vi "EventLog.New(single).vi"(7 "Source (All)":T1, 8 "error in (no error)":errorcluster, 9 "Arg":variant, 10 "Message (-)":T2, 11 "Level (Info)":T3=enum."Info") -> (0 "error out":errorcluster, 2 "Translated Msg":string)   [LabVIEW 2016]
uses:
  EventLog.EventLevel.ctl
  Translator/Translator.Message.ctl
  EventLog.EventSource.ctl
  EventLog.EventGui.ctl
  EventLog.Event.ctl
  EventLog.Buffer.Action.ctl
  Global/ApplicationGlobal.vi
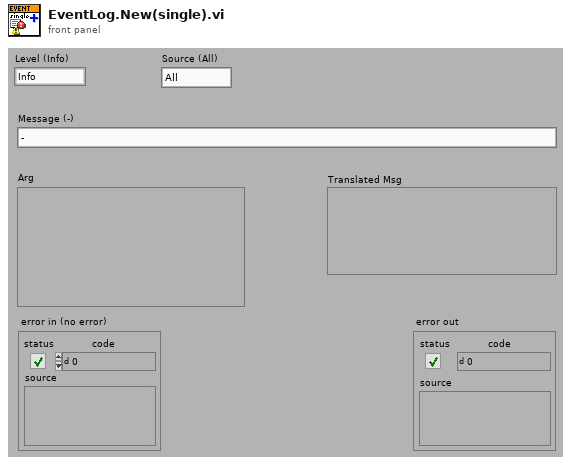
[diagram p1: front panel]
types:
  T1 = typedef "EventLog.EventSource.ctl" = enum16{"All", "Gui", "Cache", "PLC1", "PLC2", "PLC3", "DB", "DB01", "DB02", "DB03", "DB04", "DB05", "DB06", "DB07", "DB08", "DB09", "DB10", "DB11", "DB12", "DB13", "DB14", "DB15", "DB16"}
  T2 = typedef "Translator.Message.ctl" = enum16{"-", "Event confirmed", "Log out", "Log in", "Shutdown", "Cancel", "Start", "Continue", "Stop", "On", "Off", "OK", "NOK", "NOK %s", "This", "Prev", "Home", "Work", "In progress...", "Missing", "Empty", "Hardware failure", "Initial", "Error %d >> %s", "Error %d >> %s >> %s", "Starting %s", "Quitting %s", "Configured", "Initializing", "Quitting", "Loading", "Running %s", "Stopped", "Summary", "Do you want to continue?", "Do you want to exit?", "Log out?", "System", "All", "IDLE", "Translating...%s", "Not found", "Alarm %s", "Run", "Skip", "Abort", "Repeat", "Please wait...", "Database disconnected", "Login to database successful", "Login to database failed: %d; %s", "Get process step data for %s", "Changeover off", "Changeover into %s", "Product %s | %s found in cache with status %d at previous station", "Product %s | %s found in database with status %d at previous station", "Product %s | %s not found in cache at previous station", "Product %s | %s not found in database at previous station", "Product %s | %s found in cache with status %d at this station (%d repetion)", "Product %s | %s found in database with status %d at this station (%d repetition)", "Product %s | %s not found in cache at this station", "Product %s | %s not found in database at this station", "Product %s | %s found in cache for component %s | %s", "Product %s | %s found in database for component %s | %s", "Product not found in cache for component %s | %s", "Product not found in database for component %s | %s", "Product %s | %s connected with component %s | %s (cache)", "Product %s | %s connected with component %s | %s (database)", "New data for %s | %s (cache)", "New data for %s | %s (database)", "File %s moved (cache)", "File %s deleted (cache)", "Msg %d >> %s", "PLC LifeBit Failure", "Reconnecting DB", "Reconnecting PLC", "Free disk space is below 1GB - contact technician", "Unable to check product status", "Product %s SN %s checked in DB", "Unable To check status from station %s"}
  T3 = typedef "EventLog.EventLevel.ctl" = enum8{"Debug", "Info", "Warning", "Error"}
  T4 = typedef "EventLog.Event.ctl" = cluster{"ts":dbl, "lev":T3, "src":T1, "msg":T2, "arg":variant[]}
  T5 = typedef "EventLog.EventGui.ctl" = cluster{"ts":dbl, "lev":T3, "src":T1, "msg":T2, "arg":variant[], "msg_str":string}
  T6 = typedef "EventLog.Buffer.Action.ctl" = enum16{"init", "re-init", "clear", "set translator", "translate", "add", "get"}
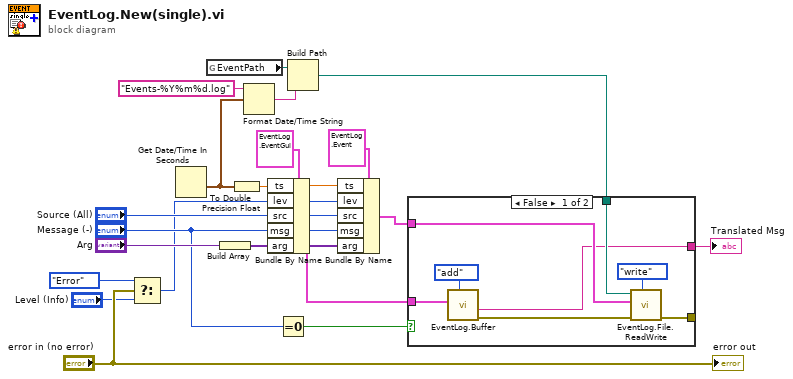
[diagram p0: block diagram]
diagram:
  n1 = Select(t=EventLog.EventLevel."Error", s="error in (no error)", f="Level (Info)") -> (s? t:f=w2:T3)
  n2 = Get Date/Time In Seconds() -> (seconds since 1Jan1904=w11:timestamp)
  n3 = global read "ApplicationGlobal.vi" "EventPath"() -> (w9:path)
  n4 = Build Array("Arg") -> (w13:variant[])
  n5 = To Double Precision Float(number=w11) -> (double precision float=w15:dbl)
  n6 = Format Date/Time String(time format string (%c)="Events-%Y%m%d.log", seconds (now)=w11) -> (date/time string=w8:string)  [unwired: 1 in]
  n7 = Bundle By Name(cluster=T5 {"ts"=0.0, "lev"=enum."Debug", "src"=enum."All", "msg"=enum."Log out", "arg"=[], "msg_str"=""} ("Event in"), "ts"=w15, "lev"=w2, "src"="Source (All)", "msg"="Message (-)", "arg"=w13) -> (w18:T5)
  n8 = Equal To 0?(x="Message (-)") -> (x = 0?=w19:bool)
  n9 = Build Path(base path=w9, name or relative path=w8) -> (appended path=w7:path)
  n10 = Bundle By Name(cluster=T4 {"ts"=0.0, "lev"=enum."Debug", "src"=enum."All", "msg"=enum."Log out", "arg"=[]} ("event in"), "ts"=w15, "lev"=w2, "src"="Source (All)", "msg"="Message (-)", "arg"=w13) -> (w12:T4)
  n11 = case shown="False" w19 {
    tunnel: w18 -> [w22 _]
    tunnel: w12 -> [w27 _]
    tunnel: w7 -> [w25 _]
    tunnel: [w24 _] -> _
    tunnel: [w23 _] -> w5
    frame False {
      n12 = call "EventLog.Buffer.vi"("action (get)"=EventLog.Buffer.Action."add" ("action (read)"), "Event in"=w22) -> ("error out"=w21:errorcluster, "Translated Msg"=w23:string)  [unwired: 6 in, 2 out]
      n13 = call "EventLog.File.ReadWrite.vi"("action (read)"=enum16{"read", "write"}."write", "error in"=w21, "event in"=w27, "file"=w25) -> ("error out"=w24:errorcluster)  [unwired: 3 in, 4 out]
    }
    frame True {
    }
  }
  "Translated Msg" <- w5
  "error out" <- "error in (no error)"
